vi "20151028 accel+gyro+kalman filter.vi"() -> ()   [LabVIEW 2013]
uses:
  <vilib>/MakerHub/LINX/Public/Sensors/Accelerometer/MPU60X0/DeviceAddresses.ctl
  <vilib>/MakerHub/LINX/Public/Sensors/Accelerometer/MPU60X0/AccelFullScaleRanges.ctl
  <vilib>/MakerHub/LINX/Public/Sensors/Accelerometer/MPU60X0/GyroFullScaleRanges.ctl
  <vilib>/MakerHub/LINX/Public/Sensors/Accelerometer/MPU60X0/MPU60X0.lvlib
  <vilib>/MakerHub/LINX/LMH-LINX.lvlib
panel:
  in  "stop":bool
  out "After kalman":cluster{"x_angle":dbl, "x_angle":dbl}(graph)
  out "roll":dbl
  out "pitch":dbl
  out "Elapsed time":u32
  out "Temperature (°C)":dbl
  out "Gyro":T1(graph)
  out "Accel":T1(graph)
  in  "Serial Port":refnum<visa-resource-name>="COM10"
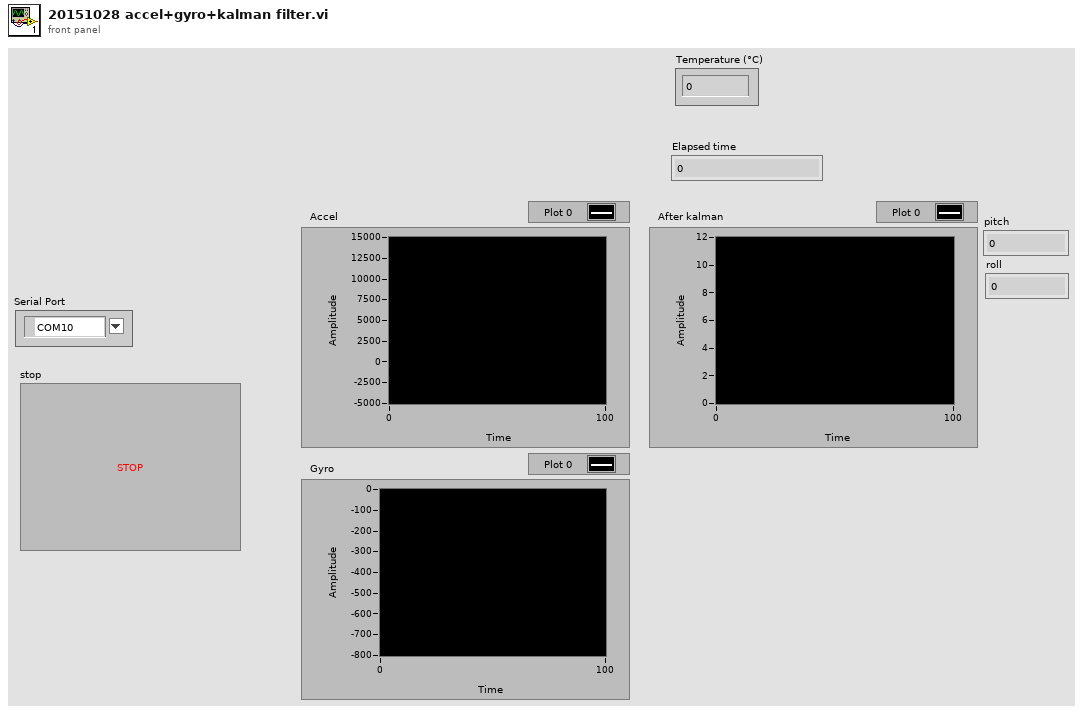
[diagram p1: front panel]
types:
  T1 = cluster{"X Axis":i16, "Y Axis":i16, "Z Axis":i16}
  T2 = typedef "LMH-LINX.lvlib/MPU60X0.lvlib/GyroFullScaleRanges.ctl" = enum8{"±250 °/s", "±500 °/s", "±1000 °/s", "±2000 °/s"}
  T3 = typedef "LMH-LINX.lvlib/MPU60X0.lvlib/AccelFullScaleRanges.ctl" = enum16{"±2g", "±4g", "±8g", "±16g"}
  T4 = typedef "LMH-LINX.lvlib/MPU60X0.lvlib/DeviceAddresses.ctl" = enum16{"0x68", "0x69"}
  T5 = typedef "LMH-LINX.lvlib/LINX Ref.ctl" = cluster{"Platform":T6, "Interface":T7, "LINX Device Config":T8}
  T6 = typedef "LMH-LINX.lvlib/Platform.ctl" = enum16{"LINX", "myRIO"}
  T7 = typedef "LMH-LINX.lvlib/Interface.ctl" = enum16{"Serial", "TCP"}
  T8 = typedef "LMH-LINX.lvlib/Device.lvlib/LINX Device Config.ctl" = cluster{"Interface":T7, "COM Port":refnum<visa-resource-name>, "TCP Configuration":T9, "Device Family":u8, "Device ID":u8, "Device Name":string, "TCP Ref":refnum<k5>, "Channels":T10}
  T9 = typedef "LMH-LINX.lvlib/Device.lvlib/TCP Config.ctl" = cluster{"IP Address":string, "Port":u16}
  T10 = typedef "LMH-LINX.lvlib/Channels.ctl" = cluster{"DI":u8[], "DO":u8[], "AI":u8[], "AO":u8[], "PWM":u8[], "QE":u8[], "UART":u8[], "I2C 2":u8[], "SPI":u8[], "CAN":u8[], "Servo":u8[], "AI Ref (V)":dbl, "AO Ref (V)":dbl, "AO Resolution (Bits)":u8}
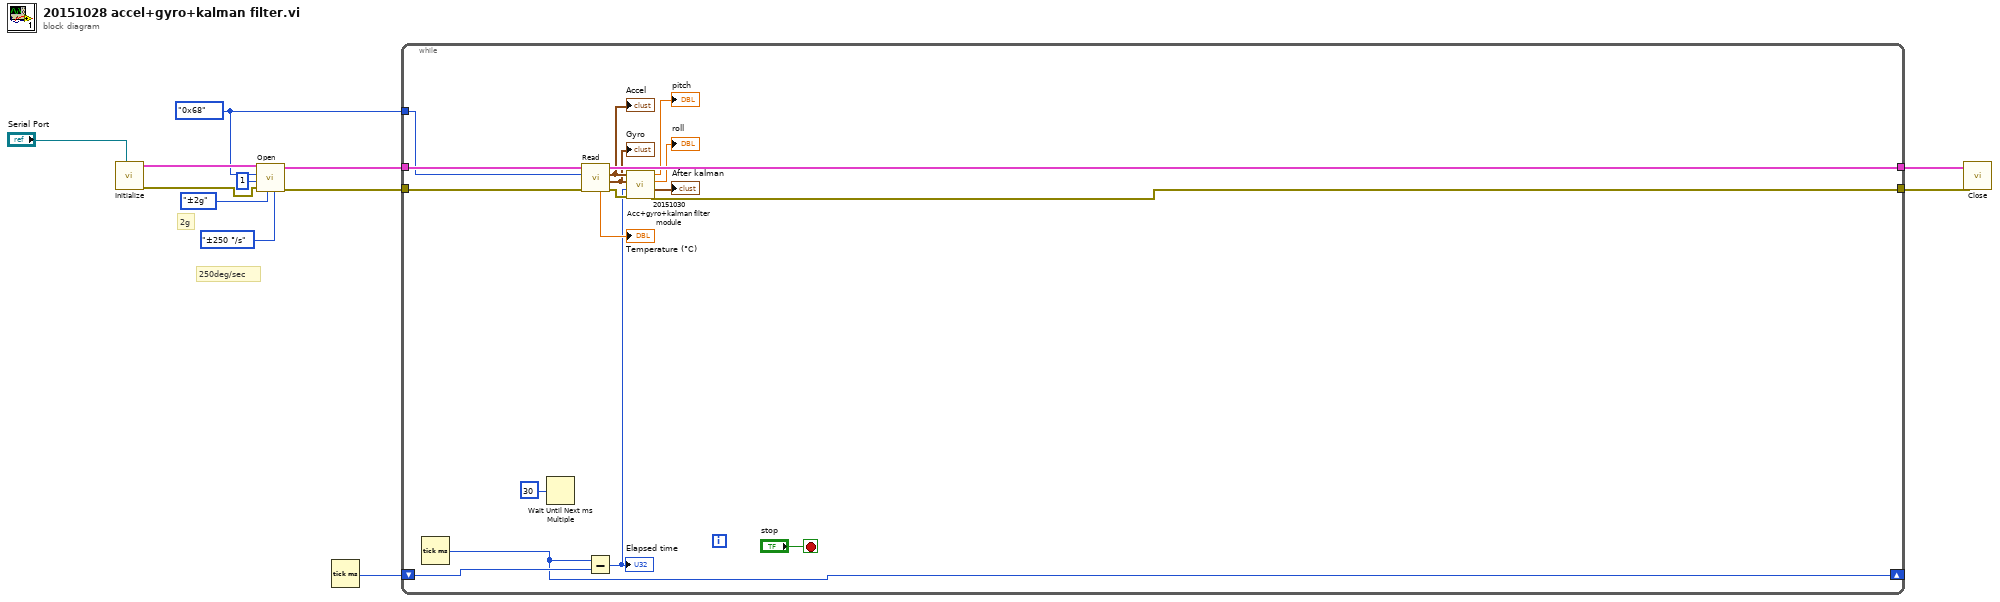
[diagram p0: block diagram]
diagram:
  w7 = DeviceAddresses."0x68" ("Device Address")
  # "250deg/sec"
  # "2g"
  n1 = call <vilib>:"Initialize.vi"("Serial Port"="Serial Port") -> ("Error Out"=w9:errorcluster, "LINX Ref"=w10:T5)  [unwired: 8 in, 1 out]
  n2 = call <vilib>:"Open.vi"("Gyro Full Scale Range"=GyroFullScaleRanges."±250 °/s", "Accel Full Scale Range"=AccelFullScaleRanges."±2g", "Error In"=w9, "Clock Source"=u8 1, "Device Address"=w7, "LINX Resource"=w10) -> ("Error Out"=w11:errorcluster, "LINX Resource"=w12:T5)  [unwired: 4 in]
  n3 = Tick Count (ms)() -> (millisecond timer value=w2:u32)
  n4 = while {
    tunnel: w12 -> [w29]
    tunnel: w11 -> [w28]
    tunnel: [w27] -> w6
    tunnel: [w19] -> w5
    tunnel: w7 -> [w26]
    shift-right: [w21] -> _
    shift-left: w2 -> [w22]
    stop <- "stop" stop-if-true
    n5 = Tick Count (ms)() -> (millisecond timer value=w21:u32)
    n6 = Wait Until Next ms Multiple(millisecond multiple=u32 30) -> ()  [unwired: 1 out]
    n7 = call <vilib>:"Read.vi"("Error In"=w28, "Device Address"=w26, "LINX Resource"=w29) -> ("Error Out"=w20:errorcluster, "Gyro  Data"=w24:T1, "Acceleration Data"=w25:T1, "LINX Resource"=w27:T5, "Temperature (°C)"=→"Temperature (°C)":dbl)  [unwired: 4 in]
    "Accel" <- w25
    "Gyro" <- w24
    n8 = Subtract(x=w21, y=w22) -> (x-y=w18:u32)
    "Elapsed time" <- w18
    n9 = call "20151030 Acc+gyro+kalman filter module.vi"("error in (no error)"=w20, "Looptime"=w18, "Gyro  Data"=w24, "Acceleration Data"=w25) -> ("error out"=w19:errorcluster, "After Kalman filter"=→"After kalman":cluster{"x_angle":dbl, "x_angle":dbl}, "roll"=→"roll":dbl, "pitch"=→"pitch":dbl)  [unwired: 4 in]
  }
  n10 = call <vilib>:"Close.vi"("Error In"=w5, "LINX Resource"=w6) -> ()  [unwired: 8 in, 2 out]
